vi "Minesweeper Drawing Engine.vi"(8 "Error In":errorcluster, 10 "GridData":T1[][](array[typedef]), 11 "Event Registration Refnum":refnum<event-registration>) -> (0 "Error Out":errorcluster, 2 "Minefield Picture Out":picture, 3 "Event Registration Refnum Out":refnum<event-registration>)   [LabVIEW 2011]
uses:
  MineSpace.ctl
  Minesweeper Drawing Event Type Def.ctl
  Minesweeper Drawing Operation Type Def.ctl
  Cover Operation Typdef.ctl
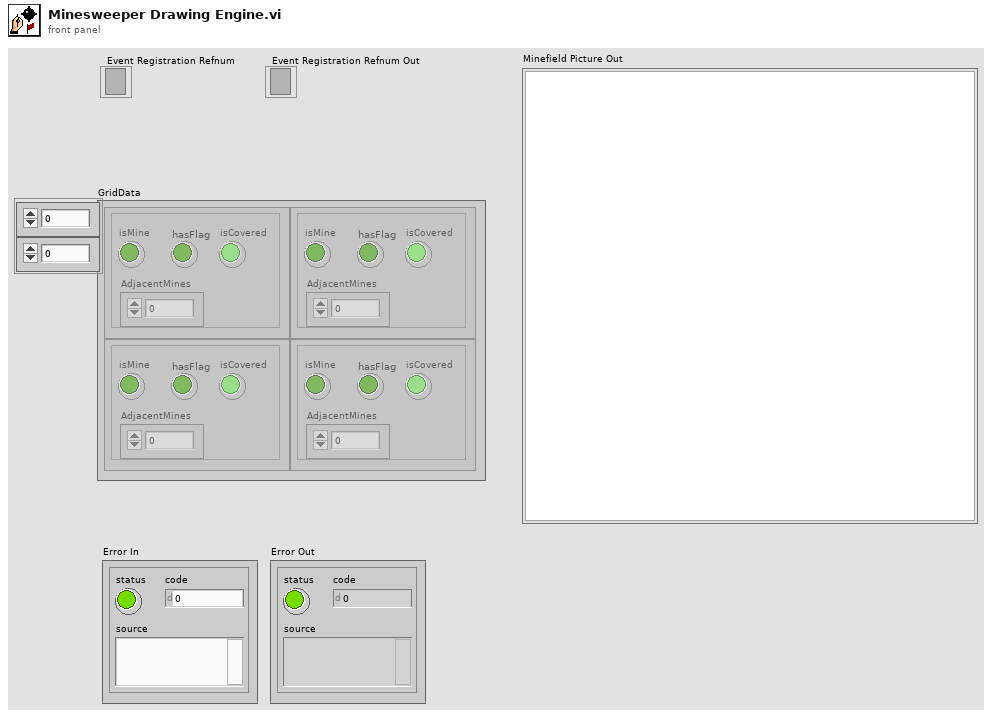
[diagram p1: front panel]
types:
  T1 = typedef "MineSpace.ctl" = cluster{"isMine":bool, "hasFlag":bool, "isCovered":bool, "AdjacentMines":u32}
  T2 = typedef "Cover Operation Typdef.ctl" = enum16{"Cover", "Uncover", "Flag", "Unflag"}
  T3 = typedef "Minesweeper Drawing Operation Type Def.ctl" = enum16{"Initialize", "Uncover", "Flag", "Unflag"}
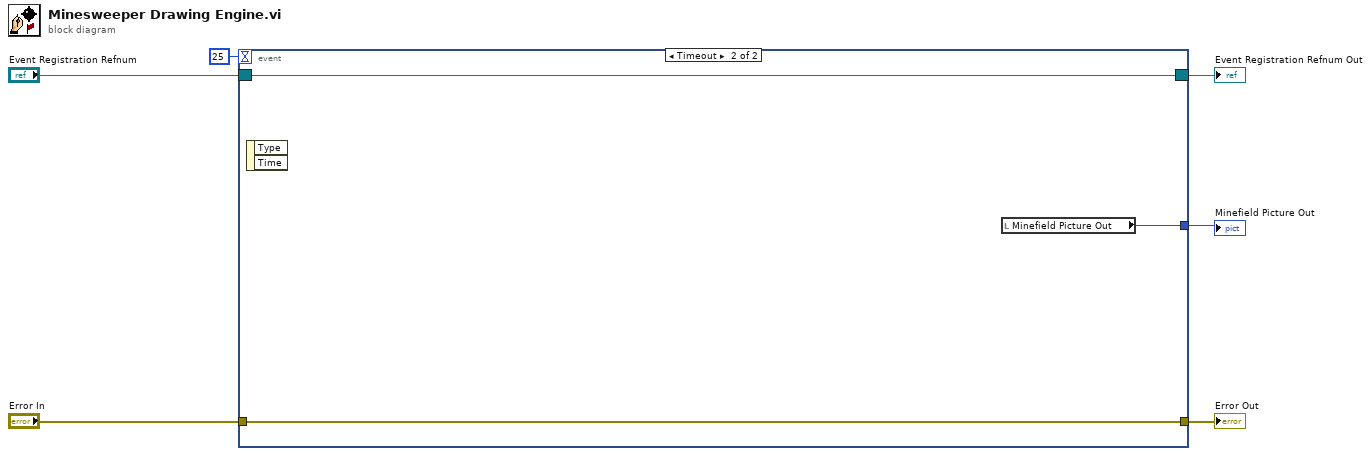
[diagram p0: block diagram]
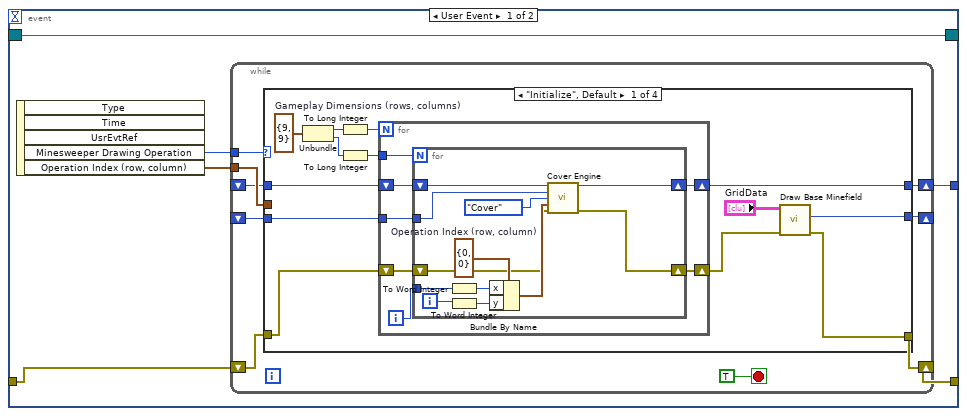
[diagram p2: hidden frame]
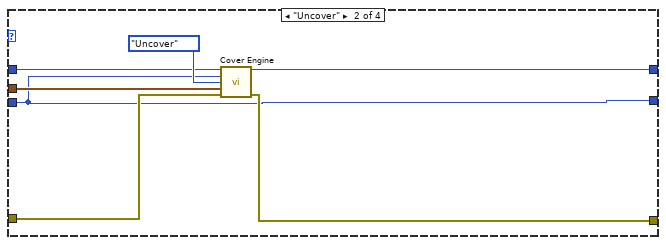
[diagram p3: hidden frame]
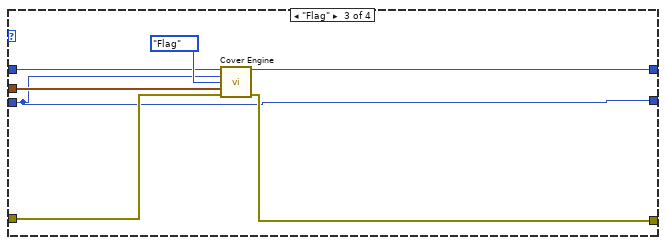
[diagram p4: hidden frame]
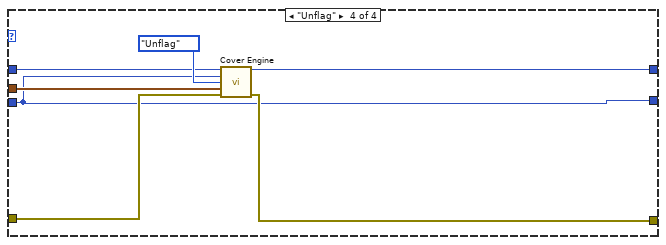
[diagram p5: hidden frame]
diagram:
  n1 = event shown="[1] Timeout" {
    selector: "Event Registration Refnum" -> [w10 w77]
    dyn-events: [w10 w77] -> w3
    timeout: 25 -> [_ _]
    tunnel: [w7 w76] -> w2
    tunnel: [w9 w75] -> w4
    tunnel: "Error In" -> [w8 w76]
    event User Event {
      n2 = event-data() -> ("Minesweeper Drawing Operation"=w12:T3, "Operation Index (row, column)"=w11:cluster{"x":i16, "y":i16})  [unwired: 1 in, 3 out]
      n3 = while {
        tunnel: w12 -> [w21]
        tunnel: w11 -> [w19]
        shift-right: [w14] -> w7
        shift-left: w8 -> [w17]
        shift-right: [w18] -> w9
        shift-left: _ -> [w15]
        shift-right: [w13] -> _
        shift-left: _ -> [w20]
        stop <- TRUE stop-if-true
        n4 = case shown="\"Initialize\", Default" w21 {
          tunnel: w20 -> [w28 w55 w62 w68]
          tunnel: w19 -> [_ w59 w66 w73]
          tunnel: [w29 w57 w64 w71] -> w18
          tunnel: [w23 w58 w65 w72] -> w14
          tunnel: w17 -> [w27 w56 w63 w70]
          tunnel: w15 -> [w26 w54 w61 w69]
          tunnel: [w25 w55 w62 w68] -> w13
          frame "Initialize", Default {
            w34 = cluster{"x":i16, "y":i16} {"x"=9, "y"=9}  # Gameplay Dimensions (rows, columns)
            n5 = Unbundle(w34) -> ("x"=w32:i16, "y"=w31:i16)
            n6 = To Long Integer(number=w32) -> (32bit integer=w33:i32)
            n7 = To Long Integer(number=w31) -> (32bit integer=w30:i32)
            n8 = for {
              N: w33 -> [_]
              tunnel: w30 -> [w41]
              tunnel: w28 -> [w39]
              shift-right: [w37] -> w24
              shift-left: w27 -> [w38]
              shift-right: [w36] -> w29
              shift-left: w26 -> [w35]
              i -> [w40]
              n9 = for {
                N: w41 -> [_]
                tunnel: w40 -> [w50]
                tunnel: w39 -> [w47]
                shift-right: [w44] -> w37
                shift-left: w38 -> [w45]
                shift-right: [w43] -> w36
                shift-left: w35 -> [w42]
                i -> [w49]
                w53 = cluster{"x":i16, "y":i16} {"x"=0, "y"=0}  # Operation Index (row, column)
                n10 = To Word Integer(number=w50) -> (16bit integer=w52:i16)
                n11 = To Word Integer(number=w49) -> (16bit integer=w51:i16)
                n12 = Bundle By Name(cluster=w53, "x"=w52, "y"=w51) -> (w48:cluster{"x":i16, "y":i16})
                n13 = call "Cover Engine.vi"("Current Minefield"=w42, "Minefield Base Picture"=w47, "Cover Operation"=Cover_Operation_Typdef."Cover", "Operation Index (row, column)"=w48, "Error In"=w45) -> ("Minefield Picture Out"=w43:picture, "Error Out"=w44:errorcluster)  [unwired: 9 in]
              }
            }
            n14 = call "Draw Base Minefield.vi"("Error In"=w24, "Grid Data"="GridData") -> ("Error Out"=w23:errorcluster, "Base Minefield Picture"=w25:picture)  [unwired: 8 in]
          }
          frame "Uncover" {
            n15 = call "Cover Engine.vi"("Current Minefield"=w54, "Minefield Base Picture"=w55, "Cover Operation"=Cover_Operation_Typdef."Uncover", "Operation Index (row, column)"=w59, "Error In"=w56) -> ("Minefield Picture Out"=w57:picture, "Error Out"=w58:errorcluster)  [unwired: 9 in]
          }
          frame "Flag" {
            n16 = call "Cover Engine.vi"("Current Minefield"=w61, "Minefield Base Picture"=w62, "Cover Operation"=Cover_Operation_Typdef."Flag", "Operation Index (row, column)"=w66, "Error In"=w63) -> ("Minefield Picture Out"=w64:picture, "Error Out"=w65:errorcluster)  [unwired: 9 in]
          }
          frame "Unflag" {
            n17 = call "Cover Engine.vi"("Current Minefield"=w69, "Minefield Base Picture"=w68, "Cover Operation"=Cover_Operation_Typdef."Unflag", "Operation Index (row, column)"=w73, "Error In"=w70) -> ("Minefield Picture Out"=w71:picture, "Error Out"=w72:errorcluster)  [unwired: 9 in]
          }
        }
      }
    }
    event Timeout {
      n18 = event-data() -> ()  [unwired: 1 in, 2 out]
      n19 = local read "Minefield Picture Out"() -> (w75:picture)
    }
  }
  "Minefield Picture Out" <- w4
  "Event Registration Refnum Out" <- w3
  "Error Out" <- w2
